vi "Write target type.vi"(8 "error in":errorcluster, 10 "hardware class":string, 11 "PL_Target Configuration in":refnum<class "PL_Target Configuration.lvclass">) -> (0 "error out":errorcluster, 3 "PL_Target Configuration out":refnum<class "PL_Target Configuration.lvclass">)   [LabVIEW 2013, in "PL_Target Configuration.lvclass"]
uses:
  PL_Target Configuration.lvclass
  PL_Target Configuration.lvclass/PL_Target Configuration.ctl
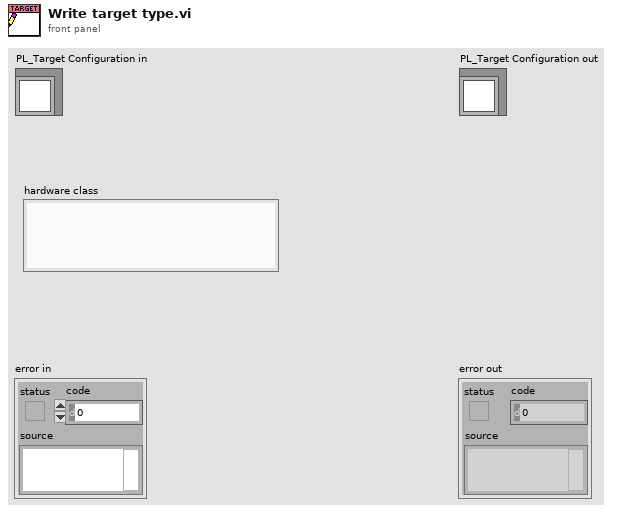
[diagram p1: front panel]
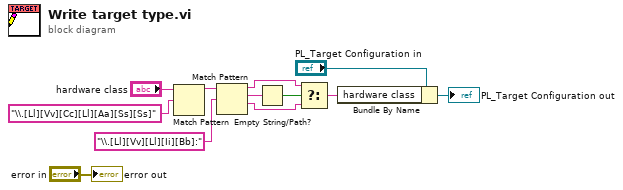
[diagram p0: block diagram]
diagram:
  n1 = Match Pattern(string="hardware class", regular expression="\\.[Ll][Vv][Cc][Ll][Aa][Ss][Ss]") -> (before substring=w7:string)  [unwired: 1 in, 3 out]
  n2 = Match Pattern(string=w7, regular expression="\\.[Ll][Vv][Ll][Ii][Bb]:") -> (before substring=w3:string, match substring=w5:string, after substring=w2:string)  [unwired: 1 in, 1 out]
  n3 = Empty String/Path?(string/path=w5) -> (empty?=w4:bool)
  n4 = Select(t=w3, s=w4, f=w2) -> (s? t:f=w1:string)
  n5 = Bundle By Name(cluster="PL_Target Configuration in", "hardware class"=w1) -> (→"PL_Target Configuration out":refnum<class "PL_Target Configuration.lvclass">)
  "error out" <- "error in"
